vi "PassOrFail (SubVI).vi"(5 "Test#":string, 6 "String Res":string, 7 "index (row)":i32, 8 "error in (no error)":errorcluster, 9 "Data in":dbl format="%#_13g", 10 "Pass?Fail":bool, 11 "Table in":refnum<vi>) -> (0 "error out":errorcluster)   [LabVIEW 2017]
uses:
  <vilib>/Utility/miscctls.llb/LVRowAndColumnTypeDef.ctl
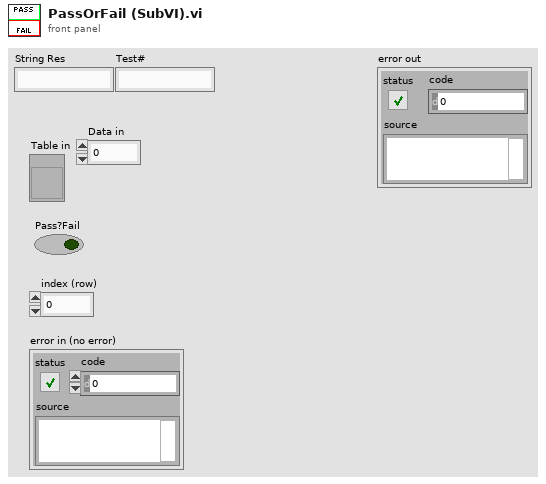
[diagram p1: front panel]
types:
  T1 = typedef "LVRowAndColumnTypeDef.ctl" = cluster{"Row":i32, "Column":i32}
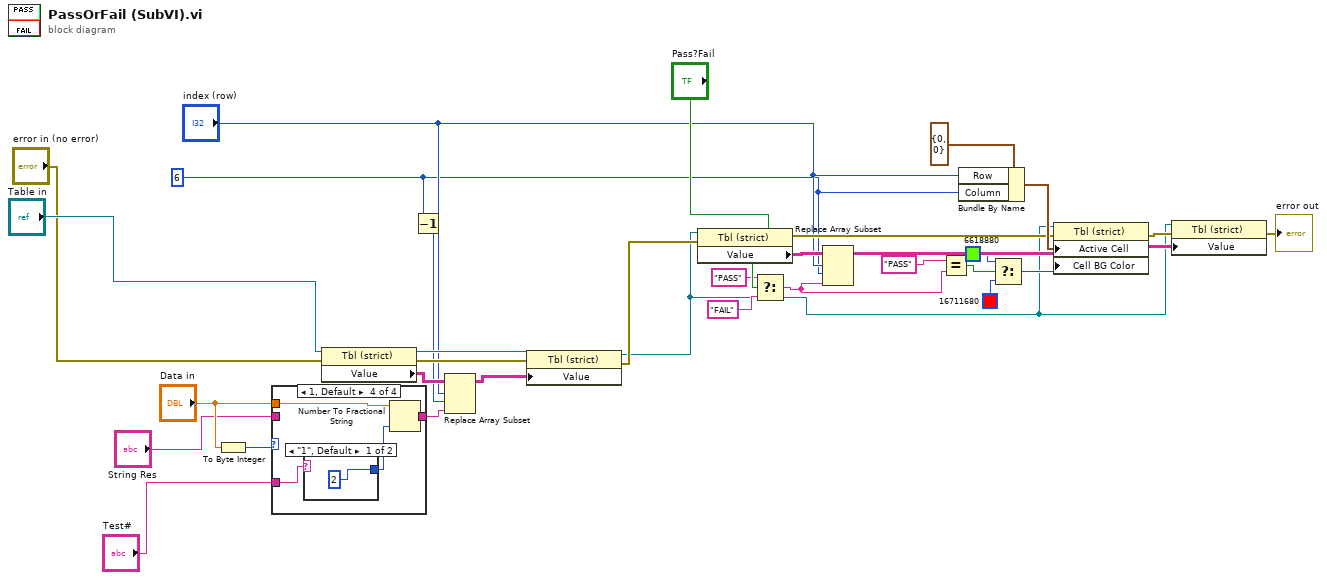
[diagram p0: block diagram]
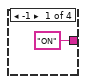
[diagram p2: hidden frame]
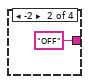
[diagram p3: hidden frame]
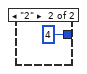
[diagram p5: hidden frame]
diagram:
  w6 = 6 ("disabled index (col)")
  n1 = To Byte Integer(number="Data in") -> (8bit integer=w3:i8)
  n2 = case shown="1, Default" w3 {
    tunnel: ["ON" "OFF" w35 w39] -> w8
    tunnel: "Data in" -> [_ _ _ w37]
    tunnel: "String Res" -> [_ _ w35 _]
    tunnel: "Test#" -> [_ _ _ w36]
    frame -1 {
    }
    frame -2 {
    }
    frame -3 {
    }
    frame 1, Default {
      n3 = case shown="\"1\", Default" w36 {
        tunnel: [i16 2 ("precision (6)") i16 4 ("precision (6)")] -> w38
        frame "1", Default {
        }
        frame "2" {
        }
      }
      n4 = Number To Fractional String(number=w37, precision (6)=w38) -> (F-format string=w39:string)  [unwired: 2 in]
    }
  }
  n5 = property class="Tbl (strict)"(reference="Table in", error in="error in (no error)") -> (reference out=w10:refnum<vi>, error out=w12:errorcluster, "Value"=w16:string[][])
  n6 = Decrement(x=w6) -> (x-1=w5:i32)
  n7 = Replace Array Subset(array=w16, new element=w8, index (row)="index (row)", index (col)=w5) -> (w15:string[][])
  n8 = property class="Tbl (strict)"(reference=w10, error in=w12, "Value"=w15) -> (reference out=w9:refnum<vi>, error out=w11:errorcluster)
  n9 = property class="Tbl (strict)"(reference=w9, error in=w11) -> (error out=w26:errorcluster, "Value"=w23:string[][])  [unwired: 1 out]
  n10 = Select(t="PASS" ("x"), s="Pass?Fail", f="FAIL" ("x")) -> (s? t:f=w29:string)
  n11 = Replace Array Subset(array=w23, new element=w29, index (row)="index (row)", index (col)=w6) -> (w24:string[][])
  n12 = Equal?(x="PASS", y=w29) -> (x = y?=w18:bool)
  n13 = Bundle By Name(cluster=T1 {"Row"=0, "Column"=0} ("Active Cell:Active Cell"), "Row"="index (row)", "Column"=w6) -> (w32:T1)
  n14 = Select(t=u32 6618880, s=w18, f=u32 16711680) -> (s? t:f=w22:u32)
  n15 = property class="Tbl (strict)"(reference=w9, error in=w26, "Active Cell"=w32, "Cell BG Color"=w22) -> (error out=w25:errorcluster)  [unwired: 1 out]
  n16 = property class="Tbl (strict)"(reference=w9, error in=w25, "Value"=w24) -> (error out=→"error out":errorcluster)  [unwired: 1 out]
